vi "FiterCheckSend.vi"(10 "TraceData":string[][](array[string]), 11 "TAFTraceWindow in":refnum<class "TAFTraceWindow.lvclass">) -> ()   [LabVIEW 2021, in "TAFTraceWindow.lvclass"]
uses:
  TAFTraceWindow.lvclass
  C:/Localdata/Projects/TriekselSoft/TriekselsoftApplicationFramework/Source/.Externals/Library_YAF/YActor/YActor.lvclass
  TAFTraceWindow.lvclass/TAFTraceWindow.ctl
  Library_YAF/YActor/YActor.lvclass
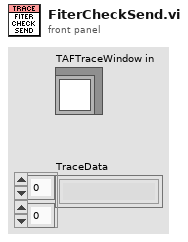
[diagram p1: front panel]
types:
  T1 = typedef "TAFTraceWindow.lvclass/FilterConfiguration.ctl" = cluster{"TraceColumn":i32, "FilterFunction":T2, "SearchText":string}
  T2 = typedef "TAFTraceWindow.lvclass/FilterFunction.ctl" = enum16{"Exact", "Regex"}
  T3 = cluster{"Name":string, "TargetQueue":refnum<queue>, "Configs":T1[]}[]
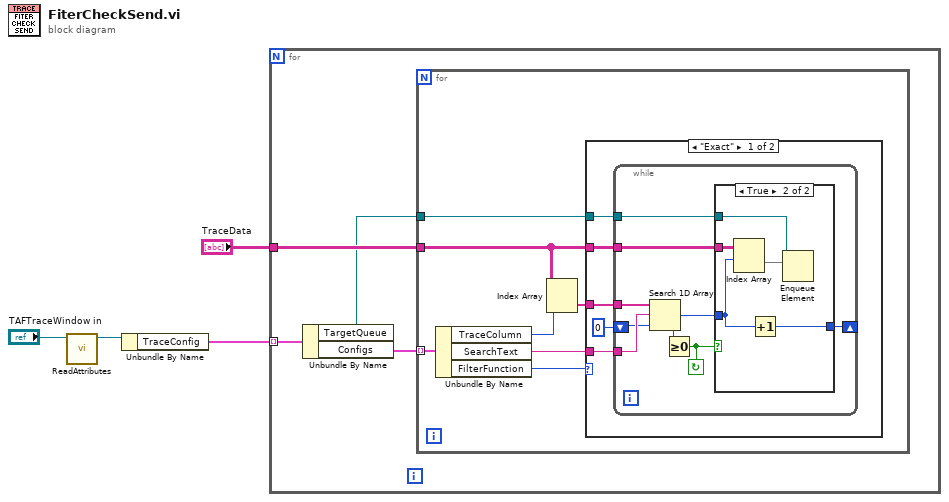
[diagram p0: block diagram]
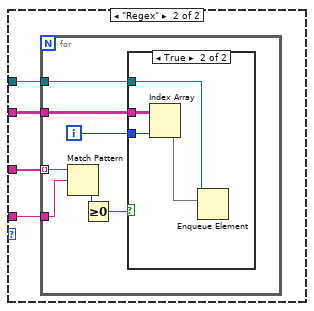
[diagram p3: hidden frame]
diagram:
  n1 = call "ReadAttributes.vi"("YActorIn"="TAFTraceWindow in") -> ("YActorOut"=w2:refnum<class "TAFTraceWindow.lvclass">)  [unwired: 9 in, 1 out]
  n2 = Unbundle By Name(w2) -> ("TraceConfig"=w1:T3)
  n3 = for {
    tunnel: "TraceData" -> [w8]
    tunnel: w1 -> [w5] mode=indexing
    n4 = Unbundle By Name(w5) -> ("TargetQueue"=w6:refnum<queue>, "Configs"=w7:T1[])
    n5 = for {
      tunnel: w7 -> [w15] mode=indexing
      tunnel: w8 -> [w10]
      tunnel: w6 -> [w9]
      n6 = Unbundle By Name(w15) -> ("TraceColumn"=w14:i32, "SearchText"=w11:string, "FilterFunction"=w13:T2)
      n7 = Index Array(array=w10, index (col)=w14) -> (element=w12:string[])  [unwired: 1 in]
      n8 = case shown="\"Exact\"" w13 {
        tunnel: w12 -> [w20 w38]
        tunnel: w11 -> [w19 w37]
        tunnel: w10 -> [w18 w36]
        tunnel: w9 -> [w17 w35]
        frame "Exact" {
          n9 = while {
            tunnel: w20 -> [w28]
            tunnel: w19 -> [w27]
            tunnel: w18 -> [w25]
            tunnel: w17 -> [w23]
            shift-right: [w22] -> _
            shift-left: 0 -> [w21]
            stop <- w26 continue-if-true
            n10 = Search 1D Array(1D array=w28, element=w27, start index (0)=w21) -> (index of element=w24:i32)
            n11 = Greater Or Equal To 0?(x=w24) -> (x >= 0?=w26:bool)
            n12 = case shown="True" w26 {
              tunnel: w25 -> [_ w33]
              tunnel: w24 -> [w29 w31]
              tunnel: w23 -> [_ w32]
              tunnel: [w29 w30] -> w22
              frame False {
              }
              frame True {
                n13 = Index Array(array=w33, index (row)=w31) -> (element=w34:string[])  [unwired: 1 in]
                n14 = Increment(x=w31) -> (x+1=w30:i32)
                n15 = Enqueue Element(queue=w32, element=w34) -> ()  [unwired: 2 in, 3 out]
              }
            }
          }
        }
        frame "Regex" {
          n16 = for {
            tunnel: w38 -> [w45] mode=indexing
            tunnel: w37 -> [w44]
            tunnel: w36 -> [w43]
            tunnel: w35 -> [w39]
            i -> [w42]
            n17 = Match Pattern(string=w45, regular expression=w44) -> (offset past match=w41:i32)  [unwired: 1 in, 3 out]
            n18 = Greater Or Equal To 0?(x=w41) -> (x >= 0?=w40:bool)
            n19 = case shown="True" w40 {
              tunnel: w43 -> [_ w49]
              tunnel: w42 -> [_ w48]
              tunnel: w39 -> [_ w46]
              frame False {
              }
              frame True {
                n20 = Index Array(array=w49, index (col)=w48) -> (element=w47:string[])  [unwired: 1 in]
                n21 = Enqueue Element(queue=w46, element=w47) -> ()  [unwired: 2 in, 3 out]
              }
            }
          }
        }
      }
    }
  }
